vi "RS触发器 (1).vi"(1 "R":bool, 2 "S":bool) -> (0 "OUT":bool)   [LabVIEW 2016]
doc: "置位和复位"
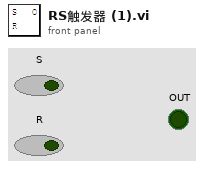
[diagram p1: front panel]
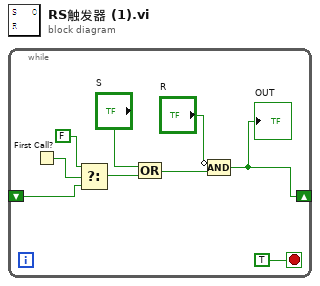
[diagram p0: block diagram]
diagram:
  n1 = while {
    shift-right: [w4] -> _
    shift-left: _ -> [w7]
    stop <- TRUE stop-if-true
    n2 = First Call?() -> (First Call?: T/F=w9:bool)
    n3 = Select(t=FALSE, s=w9, f=w7) -> (s? t:f=w6:bool)
    n4 = Compound Arithmetic op=OR("S", w6) -> (w5:bool)
    n5 = Compound Arithmetic op=AND(invert "R", w5) -> (w4:bool)
    "OUT" <- w4
  }
